vi "1.vi"() -> ()   [LabVIEW 2018]
panel:
  out "return value":dbl[][](array[numeric])
  in  "c":dbl
  in  "b":dbl
  in  "a":dbl
  out "error out":errorcluster
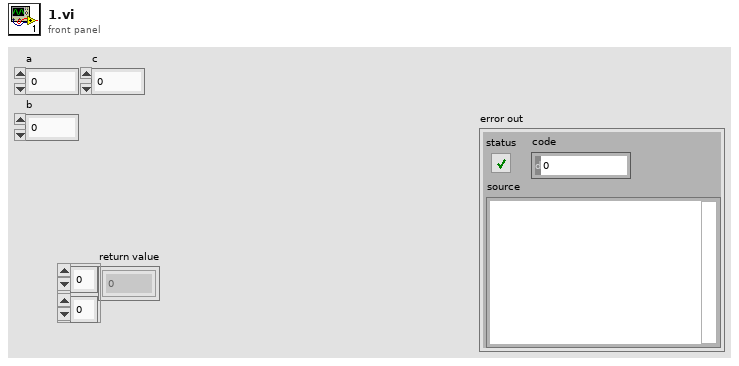
[diagram p1: front panel]
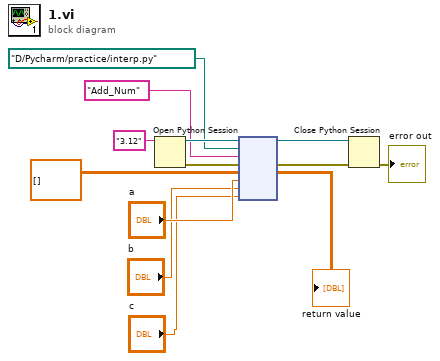
[diagram p0: block diagram]
diagram:
  n1 = Open Python Session(python version="3.12" ("Python version")) -> (session out=w13:refnum<k35>, error out=w12:errorcluster)  [unwired: 2 in]
  n2 = node(w13, path "D:/Pycharm/practice/interp.py" ("module path"), "Add_Num" ("function name"), w12, dbl[][] [] ("array"), "a", "b", "c") -> (w10:refnum<k35>, w11:errorcluster, →"return value":dbl[][])  [unwired: 3 in, 2 out]
  n3 = Close Python Session(session in=w10, error in=w11) -> (11:→"error out":errorcluster)
